vi "read log test.vi"() -> ()   [LabVIEW 2018]
uses:
  <vilib>/Utility/file.llb/Read Delimited Spreadsheet (string).vi
  subvis/Timestamp String to LV Timestamp Array.vi
panel:
  out "Waveform Graph":dbl[](graph)
  out "all rows":string[][](array[string])
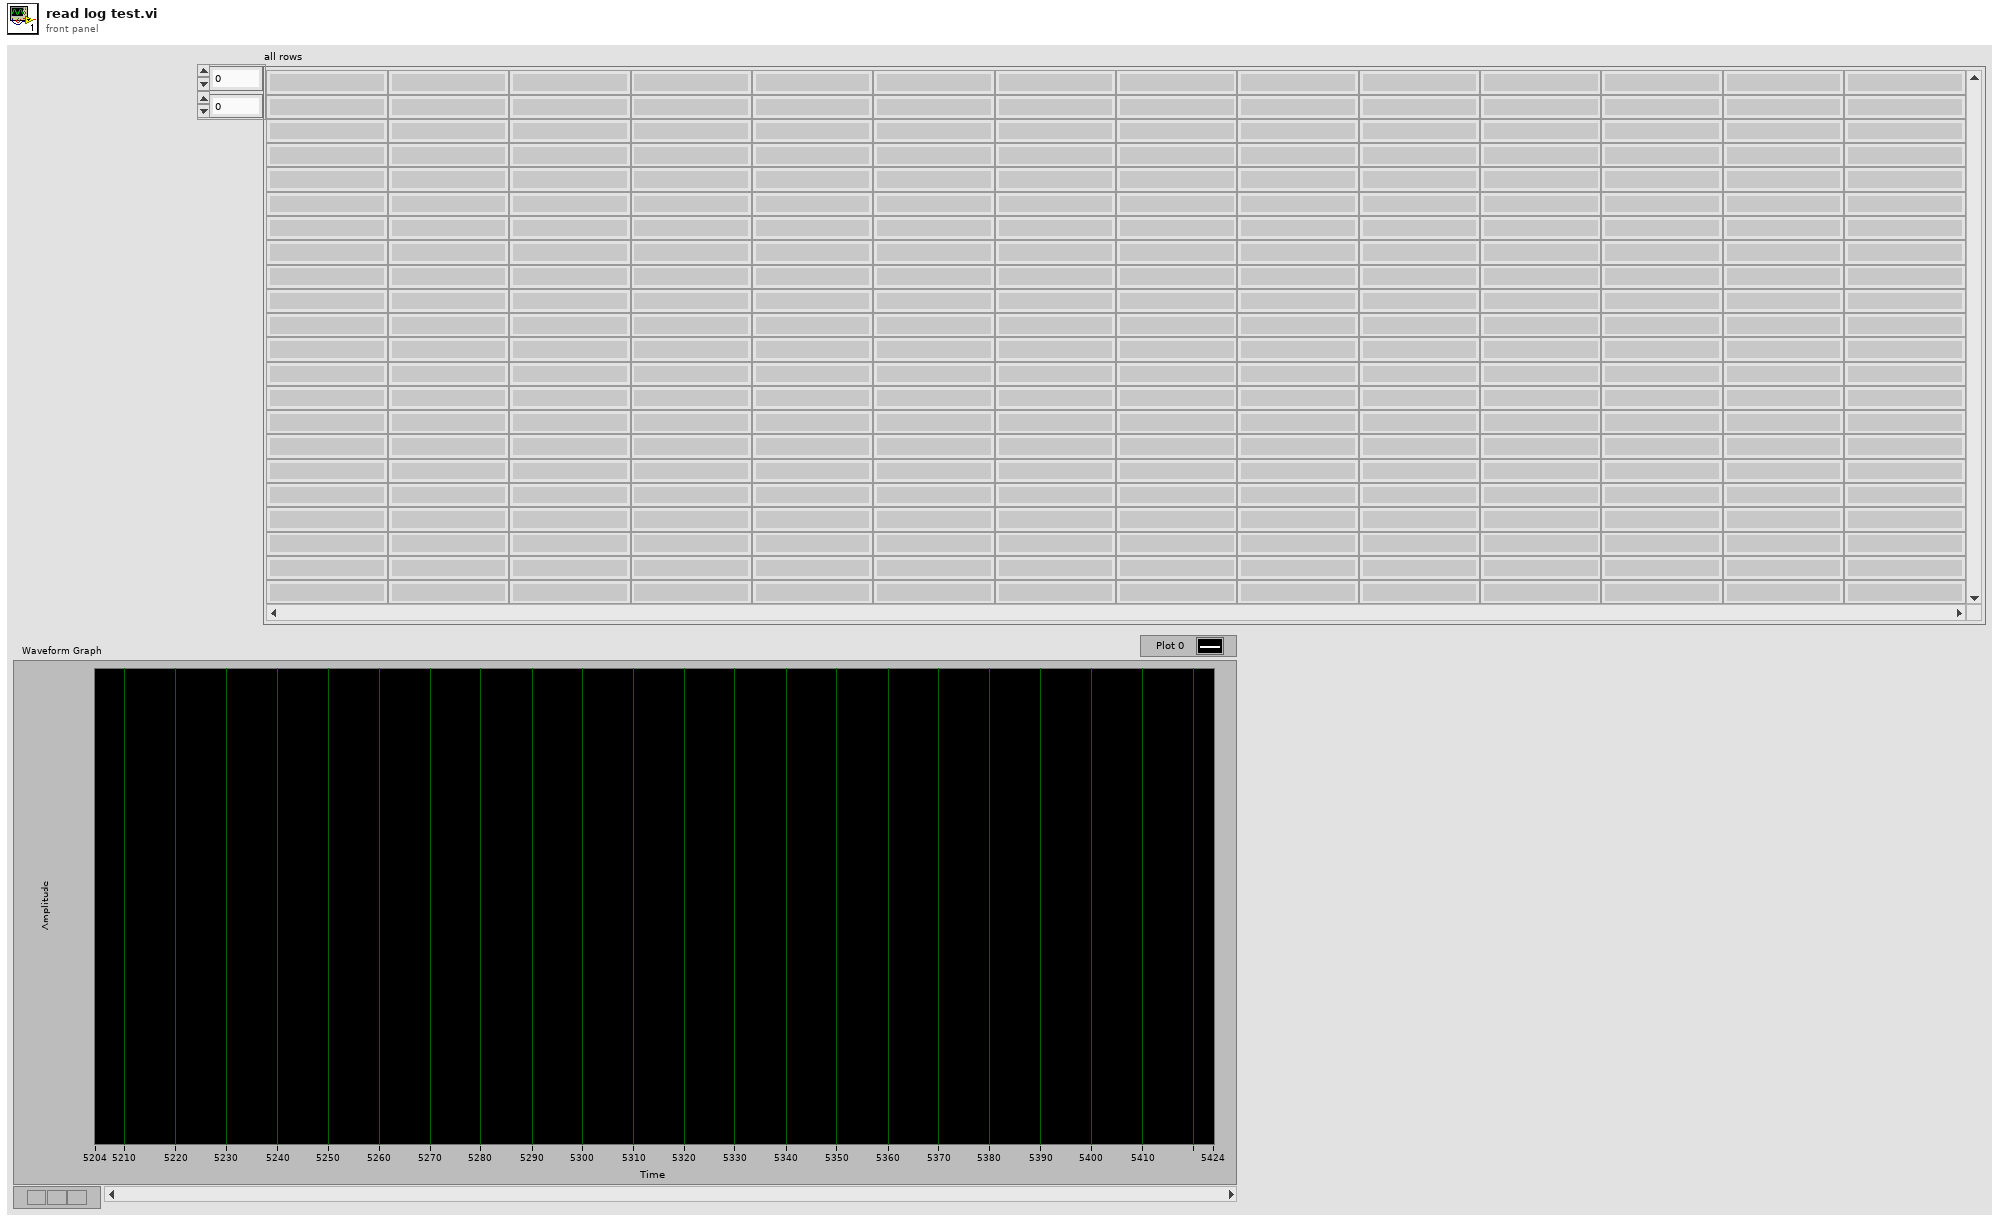
[diagram p1: front panel]
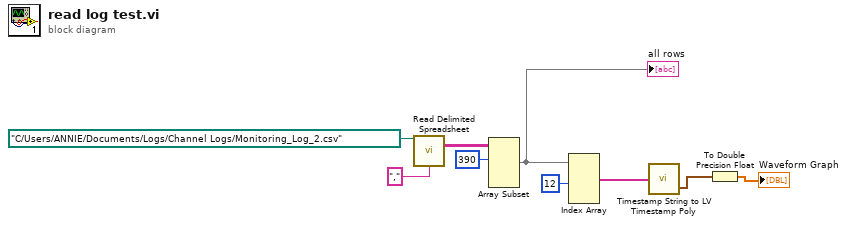
[diagram p0: block diagram]
diagram:
  n1 = call-poly <vilib>:"Read Delimited Spreadsheet.vi"("file path (dialog if empty)"=path "C:/Users/ANNIE/Documents/Logs/Channel Logs/Monitoring_Log_2.csv", "delimiter (\\t)"="," ("delimiter (\\t)")) -> ("all rows"=w7:string[][])  [unwired: 8 in, 5 out]
  n2 = Array Subset(array=w7, index (row)=390 ("index")) -> (w5:string[][])  [unwired: 3 in]
  "all rows" <- w5
  n3 = Index Array(array=w5, index (col) #1=12 ("disabled index (col)")) -> (element #1=w3:string[])  [unwired: 3 in, 1 out]
  n4 = call-poly "Timestamp String to LV Timestamp Poly.vi"("Array"=w3) -> ("Array 2"=w2:timestamp[])  [unwired: 1 out]
  n5 = To Double Precision Float(number=w2) -> (double precision float=→"Waveform Graph":dbl[])
